vi "ZZZ otro horror Chroma 1905x Series Get Hipot Configuration.vi"(0 "inst handle in":refnum<visa-resource-name>, 3 "Step Number":dbl=1.0 min=1.0 max=25.0 step=1.0, 5 "error in":T1) -> (8 "Real Current Limit":string, 9 "Test Time":string, 10 "Mode":string, 11 "Channels High":string, 12 "Voltage Level":string, 13 "Channels Low":string, 14 "inst handle out":refnum<visa-resource-name>, 15 "Hi Limit":string, 16 "Low Limit":string, 17 "Arc Detection Limit":string, 18 "Ramp Time":string, 19 "error out":T1)   [LabVIEW 2025]
doc: "Contact Chroma\nTEL: +886-2-2298-3855 \nTEL: +886-3-397-5788 \nFAX: +886-2-2298-3596\nFAX: +886-3-327-4703 \nURL: http://www.chromaate.com \nE-mail: chroma@chroma.com.tw"
panel:
  # "Get Configuration Screen"
  # "Get Hipot Configuration"
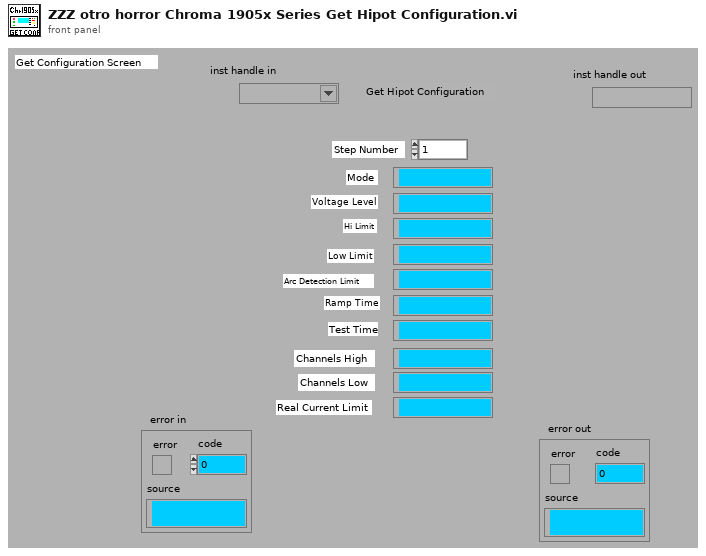
[diagram p1: front panel]
types:
  T1 = cluster{"error":bool, "code":i8, "source":string}
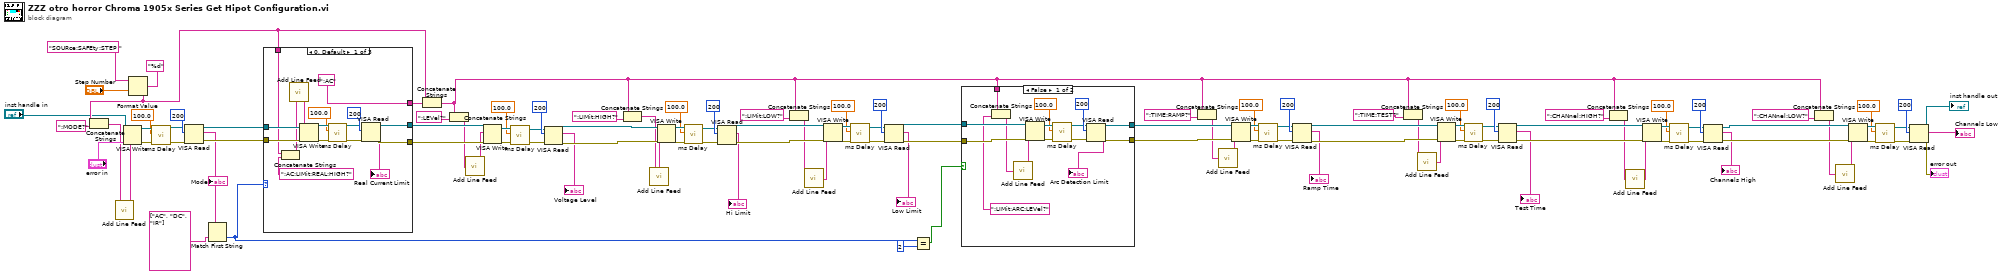
[diagram p0: block diagram]
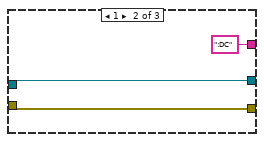
[diagram p3: hidden frame]
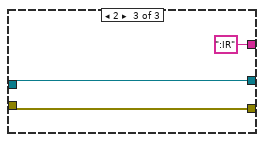
[diagram p4: hidden frame]
diagram:
  n1 = Format Value(string ("")="SOURce:SAFEty:STEP ", format string="%d", value (0)="Step Number") -> (output string=w23:string)
  n2 = Concatenate Strings(w23, ":MODE?") -> (w21:string)
  n3 = call <instrlib>:"Add Line Feed.vi"("Command string"=w21) -> ("Concatenated string"=w20:string)  [unwired: 4 in]
  n4 = VISA Write(VISA resource name="inst handle in", write buffer=w20, error in (no error)="error in") -> (VISA resource name out=w103:refnum<visa-resource-name>, error out=w106:errorcluster)  [unwired: 1 out]
  n5 = call <instrlib>:"ms Delay.vi"("error in (no error)"=w106, "Time Delay [ms]"=100.0 ("Time Delay S"), "VISA resource name"=w103) -> ("error out"=w105:errorcluster, "VISA resource name 2"=w104:refnum<visa-resource-name>)  [unwired: 7 in]
  n6 = VISA Read(VISA resource name=w104, byte count=u32 200 ("byte count (0)"), error in (no error)=w105) -> (VISA resource name out=w26:refnum<visa-resource-name>, read buffer=w5:string, error out=w27:errorcluster)  [unwired: 1 out]
  "Mode" <- w5
  n7 = Match First String(2:string[] ["AC", "DC", "IR"] ("string array"), 3:w5) -> (0:w1:i32)  [unwired: 1 out]
  n8 = case shown="0, Default" w1 {
    tunnel: [":AC" ":DC" ":IR"] -> w94
    tunnel: w27 -> [w127 w129 w132]
    tunnel: w26 -> [w126 w130 w133]
    tunnel: [w125 w130 w133] -> w25
    tunnel: [w124 w129 w132] -> w24
    tunnel: w23 -> [w123 _ _]
    frame 0, Default {
      n9 = Concatenate Strings(w123, ":AC:LIMit:REAL:HIGH?" ("write buffer (\"\")")) -> (w114:string)
      n10 = call <instrlib>:"Add Line Feed.vi"("Command string"=w114) -> ("Concatenated string"=w113:string)  [unwired: 4 in]
      n11 = VISA Write(VISA resource name=w126, write buffer=w113, error in (no error)=w127) -> (VISA resource name out=w118:refnum<visa-resource-name>, error out=w121:errorcluster)  [unwired: 1 out]
      n12 = call <instrlib>:"ms Delay.vi"("error in (no error)"=w121, "Time Delay [ms]"=100.0 ("Time Delay S"), "VISA resource name"=w118) -> ("error out"=w120:errorcluster, "VISA resource name 2"=w119:refnum<visa-resource-name>)  [unwired: 7 in]
      n13 = VISA Read(VISA resource name=w119, byte count=u32 200 ("byte count (0)"), error in (no error)=w120) -> (VISA resource name out=w125:refnum<visa-resource-name>, read buffer=→"Real Current Limit":string, error out=w124:errorcluster)  [unwired: 1 out]
    }
    frame 1 {
    }
    frame 2 {
    }
  }
  n14 = Concatenate Strings(w23, w94) -> (w35:string)
  n15 = Concatenate Strings(w35, ":LEVel?") -> (w19:string)
  n16 = call <instrlib>:"Add Line Feed.vi"("Command string"=w19) -> ("Concatenated string"=w18:string)  [unwired: 4 in]
  n17 = VISA Write(VISA resource name=w25, write buffer=w18, error in (no error)=w24) -> (VISA resource name out=w96:refnum<visa-resource-name>, error out=w99:errorcluster)  [unwired: 1 out]
  n18 = call <instrlib>:"ms Delay.vi"("error in (no error)"=w99, "Time Delay [ms]"=100.0 ("Time Delay S"), "VISA resource name"=w96) -> ("error out"=w98:errorcluster, "VISA resource name 2"=w97:refnum<visa-resource-name>)  [unwired: 7 in]
  n19 = VISA Read(VISA resource name=w97, byte count=u32 200 ("byte count (0)"), error in (no error)=w98) -> (VISA resource name out=w85:refnum<visa-resource-name>, read buffer=→"Voltage Level":string, error out=w86:errorcluster)  [unwired: 1 out]
  n20 = Concatenate Strings(w35, ":LIMit:HIGH?") -> (w7:string)
  n21 = call <instrlib>:"Add Line Feed.vi"("Command string"=w7) -> ("Concatenated string"=w6:string)  [unwired: 4 in]
  n22 = VISA Write(VISA resource name=w85, write buffer=w6, error in (no error)=w86) -> (VISA resource name out=w88:refnum<visa-resource-name>, error out=w91:errorcluster)  [unwired: 1 out]
  n23 = call <instrlib>:"ms Delay.vi"("error in (no error)"=w91, "Time Delay [ms]"=100.0 ("Time Delay S"), "VISA resource name"=w88) -> ("error out"=w90:errorcluster, "VISA resource name 2"=w89:refnum<visa-resource-name>)  [unwired: 7 in]
  n24 = VISA Read(VISA resource name=w89, byte count=u32 200 ("byte count (0)"), error in (no error)=w90) -> (VISA resource name out=w76:refnum<visa-resource-name>, read buffer=→"Hi Limit":string, error out=w77:errorcluster)  [unwired: 1 out]
  n25 = Concatenate Strings(w35, ":LIMit:LOW?") -> (w17:string)
  n26 = call <instrlib>:"Add Line Feed.vi"("Command string"=w17) -> ("Concatenated string"=w16:string)  [unwired: 4 in]
  n27 = VISA Write(VISA resource name=w76, write buffer=w16, error in (no error)=w77) -> (VISA resource name out=w79:refnum<visa-resource-name>, error out=w82:errorcluster)  [unwired: 1 out]
  n28 = call <instrlib>:"ms Delay.vi"("error in (no error)"=w82, "Time Delay [ms]"=100.0 ("Time Delay S"), "VISA resource name"=w79) -> ("error out"=w81:errorcluster, "VISA resource name 2"=w80:refnum<visa-resource-name>)  [unwired: 7 in]
  n29 = VISA Read(VISA resource name=w80, byte count=u32 200 ("byte count (0)"), error in (no error)=w81) -> (VISA resource name out=w74:refnum<visa-resource-name>, read buffer=→"Low Limit":string, error out=w75:errorcluster)  [unwired: 1 out]
  n30 = Equal?(x=w1, y=i8 2) -> (x = y?=w2:bool)
  n31 = case shown="False" w2 {
    tunnel: w75 -> [w149 w150]
    tunnel: w74 -> [w148 w151]
    tunnel: [w147 w151] -> w39
    tunnel: w35 -> [w146 _]
    tunnel: [w145 w150] -> w34
    frame False {
      n32 = Concatenate Strings(w146, ":LIMit:ARC:LEVel?") -> (w136:string)
      n33 = call <instrlib>:"Add Line Feed.vi"("Command string"=w136) -> ("Concatenated string"=w135:string)  [unwired: 4 in]
      n34 = VISA Write(VISA resource name=w148, write buffer=w135, error in (no error)=w149) -> (VISA resource name out=w139:refnum<visa-resource-name>, error out=w142:errorcluster)  [unwired: 1 out]
      n35 = call <instrlib>:"ms Delay.vi"("error in (no error)"=w142, "Time Delay [ms]"=100.0 ("Time Delay S"), "VISA resource name"=w139) -> ("error out"=w141:errorcluster, "VISA resource name 2"=w140:refnum<visa-resource-name>)  [unwired: 7 in]
      n36 = VISA Read(VISA resource name=w140, byte count=u32 200 ("byte count (0)"), error in (no error)=w141) -> (VISA resource name out=w147:refnum<visa-resource-name>, read buffer=→"Arc Detection Limit":string, error out=w145:errorcluster)  [unwired: 1 out]
    }
    frame True {
    }
  }
  n37 = Concatenate Strings(w35, ":TIME:RAMP?") -> (w15:string)
  n38 = call <instrlib>:"Add Line Feed.vi"("Command string"=w15) -> ("Concatenated string"=w14:string)  [unwired: 4 in]
  n39 = VISA Write(VISA resource name=w39, write buffer=w14, error in (no error)=w34) -> (VISA resource name out=w65:refnum<visa-resource-name>, error out=w68:errorcluster)  [unwired: 1 out]
  n40 = call <instrlib>:"ms Delay.vi"("error in (no error)"=w68, "Time Delay [ms]"=100.0 ("Time Delay S"), "VISA resource name"=w65) -> ("error out"=w67:errorcluster, "VISA resource name 2"=w66:refnum<visa-resource-name>)  [unwired: 7 in]
  n41 = VISA Read(VISA resource name=w66, byte count=u32 200 ("byte count (0)"), error in (no error)=w67) -> (VISA resource name out=w40:refnum<visa-resource-name>, read buffer=→"Ramp Time":string, error out=w38:errorcluster)  [unwired: 1 out]
  n42 = Concatenate Strings(w35, ":TIME:TEST?") -> (w13:string)
  n43 = call <instrlib>:"Add Line Feed.vi"("Command string"=w13) -> ("Concatenated string"=w12:string)  [unwired: 4 in]
  n44 = VISA Write(VISA resource name=w40, write buffer=w12, error in (no error)=w38) -> (VISA resource name out=w58:refnum<visa-resource-name>, error out=w61:errorcluster)  [unwired: 1 out]
  n45 = call <instrlib>:"ms Delay.vi"("error in (no error)"=w61, "Time Delay [ms]"=100.0 ("Time Delay S"), "VISA resource name"=w58) -> ("error out"=w60:errorcluster, "VISA resource name 2"=w59:refnum<visa-resource-name>)  [unwired: 7 in]
  n46 = VISA Read(VISA resource name=w59, byte count=u32 200 ("byte count (0)"), error in (no error)=w60) -> (VISA resource name out=w41:refnum<visa-resource-name>, read buffer=→"Test Time":string, error out=w36:errorcluster)  [unwired: 1 out]
  n47 = Concatenate Strings(w35, ":CHANnel:HIGH?") -> (w11:string)
  n48 = call <instrlib>:"Add Line Feed.vi"("Command string"=w11) -> ("Concatenated string"=w10:string)  [unwired: 4 in]
  n49 = VISA Write(VISA resource name=w41, write buffer=w10, error in (no error)=w36) -> (VISA resource name out=w51:refnum<visa-resource-name>, error out=w54:errorcluster)  [unwired: 1 out]
  n50 = call <instrlib>:"ms Delay.vi"("error in (no error)"=w54, "Time Delay [ms]"=100.0 ("Time Delay S"), "VISA resource name"=w51) -> ("error out"=w53:errorcluster, "VISA resource name 2"=w52:refnum<visa-resource-name>)  [unwired: 7 in]
  n51 = VISA Read(VISA resource name=w52, byte count=u32 200 ("byte count (0)"), error in (no error)=w53) -> (VISA resource name out=w42:refnum<visa-resource-name>, read buffer=→"Channels High":string, error out=w37:errorcluster)  [unwired: 1 out]
  n52 = Concatenate Strings(w35, ":CHANnel:LOW?") -> (w9:string)
  n53 = call <instrlib>:"Add Line Feed.vi"("Command string"=w9) -> ("Concatenated string"=w8:string)  [unwired: 4 in]
  n54 = VISA Write(VISA resource name=w42, write buffer=w8, error in (no error)=w37) -> (VISA resource name out=w44:refnum<visa-resource-name>, error out=w47:errorcluster)  [unwired: 1 out]
  n55 = call <instrlib>:"ms Delay.vi"("error in (no error)"=w47, "Time Delay [ms]"=100.0 ("Time Delay S"), "VISA resource name"=w44) -> ("error out"=w46:errorcluster, "VISA resource name 2"=w45:refnum<visa-resource-name>)  [unwired: 7 in]
  n56 = VISA Read(VISA resource name=w45, byte count=u32 200 ("byte count (0)"), error in (no error)=w46) -> (VISA resource name out=→"inst handle out":refnum<visa-resource-name>, read buffer=→"Channels Low":string, error out=→"error out":errorcluster)  [unwired: 1 out]
